vi "Full Report Dialog.vi"(9 "Time Reports In":string[](array[string]), 11 "Total Hours In":string[](array[string])) -> ()   [LabVIEW 2020]
panel:
  out "Time Reports":string[](array[string])
  out "Total Hours":string[](array[string])
  in  "Stop Button":bool
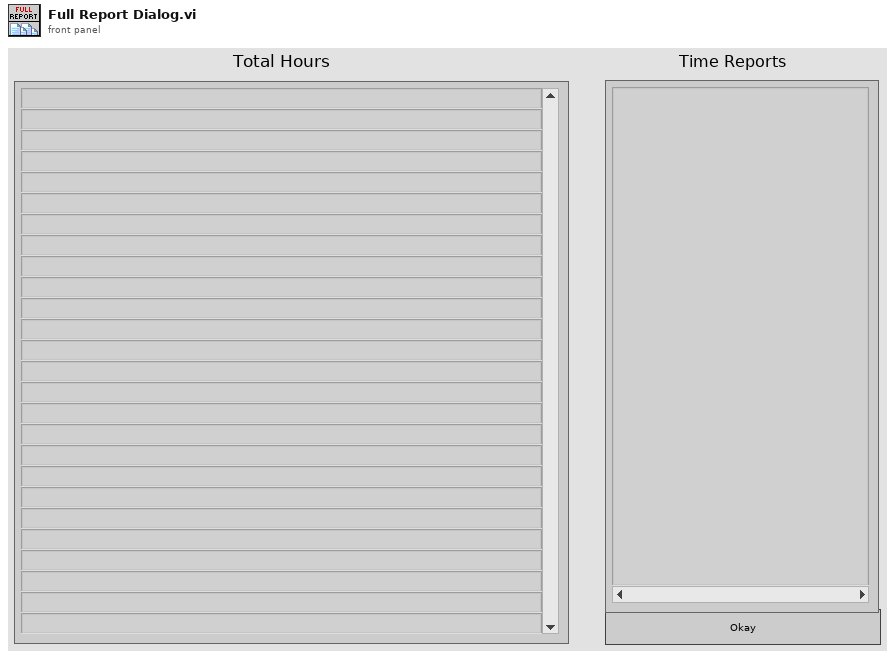
[diagram p1: front panel]
types:
  T1 = enum16{"open", "replace", "create", "open or create", "replace or create", "replace or create with confirmation"}
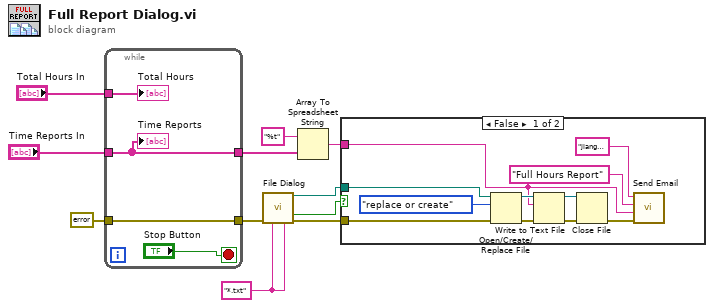
[diagram p0: block diagram]
diagram:
  w6 = "*.txt" ("pattern (all files)")
  n1 = while {
    tunnel: "Time Reports In" -> [w13]
    tunnel: "Total Hours In" -> [w14]
    tunnel: [w13] -> w9
    tunnel: [w12] -> w4
    tunnel: errorcluster {"status"=FALSE, "code"=0, "source"=""} ("error constant") -> [w12]
    stop <- "Stop Button" stop-if-true
    "Time Reports" <- w13
    "Total Hours" <- w14
  }
  n2 = call "File Dialog"("error in"=w4, "pattern (all files)"=w6, "pattern label"=w6) -> ("selected path"=w3:path, "cancelled"=w1:bool, "error out"=w5:errorcluster)  [unwired: 9 in, 1 out]
  n3 = Array To Spreadsheet String(array=w9, 3:"%t" ("format string")) -> (spreadsheet string=w2:string)  [unwired: 1 in]
  n4 = case shown="False" w1 {
    tunnel: w5 -> [w21 _]
    tunnel: w3 -> [w20 _]
    tunnel: w2 -> [w16 _]
    frame False {
      n5 = Open/Create/Replace File(file path (use dialog)=w20, error in=w21, operation (0:open)=T1."replace or create") -> (refnum out=w23:refnum<file>, error out=w26:errorcluster)  [unwired: 3 in, 1 out]
      n6 = Write to Text File(file (use dialog)=w23, text=w16, error in=w26) -> (refnum out=w24:refnum<file>, error out=w25:errorcluster)  [unwired: 1 in, 1 out]
      n7 = Close File(refnum=w24, error in=w25) -> (error out=w18:errorcluster)  [unwired: 1 out]
      n8 = call "Send Email"("error in"=w18, "Message"=w16, "Subject"="Full Hours Report", "Recipients"="jiang_voicelab@yahoo.com") -> ()  [unwired: 7 in, 1 out]
    }
    frame True {
    }
  }
